vi "Generate Simulated Data v2.0.vi"(6 "Frequency":dbl, 7 "Amplitude":dbl, 8 "error in (no error)":errorcluster, 9 "Samples":i32, 10 "Total_Samples in":i64, 11 "Sample_Rate":dbl) -> (0 "error out":errorcluster, 2 "total_samples out":i64, 3 "Y":dbl[](array[numeric]))   [LabVIEW 2026, in "Acquisition.lvlib"]
uses:
  Acquisition.lvlib
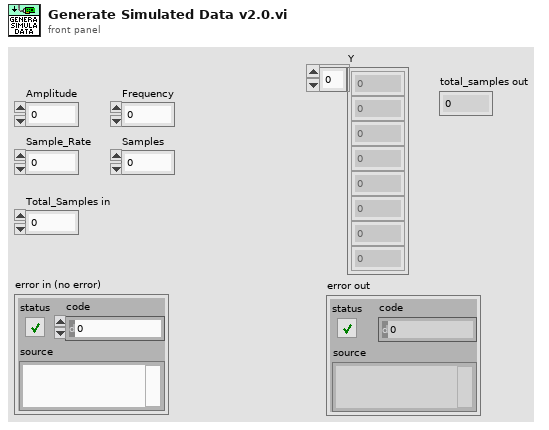
[diagram p1: front panel]
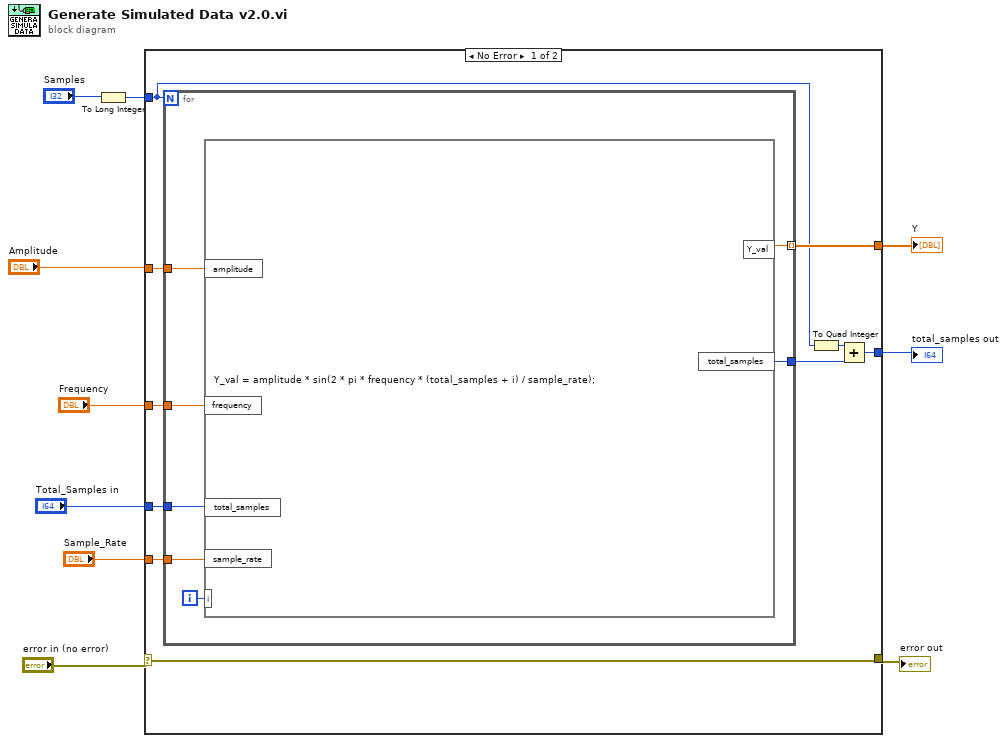
[diagram p0: block diagram]
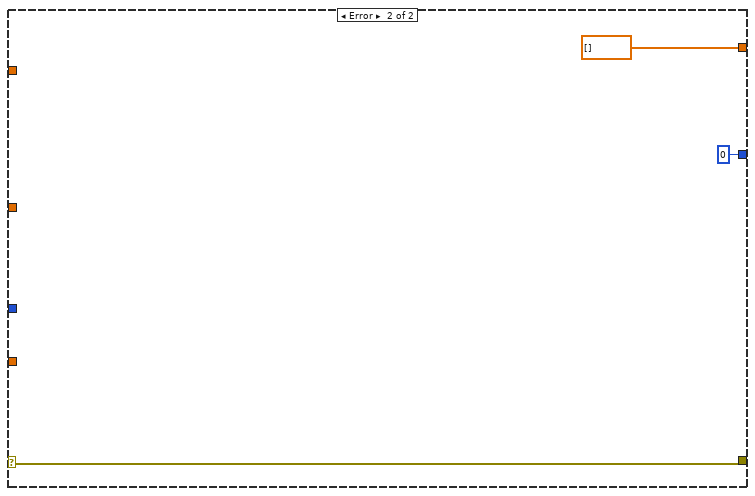
[diagram p2: hidden frame]
diagram:
  n1 = To Long Integer(number="Samples") -> (32bit integer=w2:i32)
  n2 = case shown="No Error" "error in (no error)" {
    selector: "error in (no error)" -> [w16 w30]
    tunnel: "Sample_Rate" -> [w20 _]
    tunnel: "Total_Samples in" -> [w19 _]
    tunnel: "Amplitude" -> [w18 _]
    tunnel: "Frequency" -> [w17 _]
    tunnel: [w16 w30] -> w5
    tunnel: [w15 dbl[] []] -> w4
    tunnel: w2 -> [w12 _]
    tunnel: [w11 i64 0] -> w1
    frame No Error {
      n3 = for {
        N: w12 -> [_]
        tunnel: w20 -> [w27]
        tunnel: w19 -> [w26]
        tunnel: w18 -> [w25]
        tunnel: w17 -> [w24]
        tunnel: [w23] -> w15 mode=indexing
        tunnel: [w21] -> w14
        i -> [w22]
        n4 = formula code="Y_val = amplitude * sin(2 * pi * frequency * (total_samples + i) / sample_rate);"("frequency"=w24, "amplitude"=w25, "sample_rate"=w27, "total_samples"=w26, "i"=w22) -> ("Y_val"=w23:dbl, "total_samples"=w21:i64)
      }
      n5 = To Quad Integer(1:w12) -> (0:w13:i64)
      n6 = Add(x=w13, y=w14) -> (x+y=w11:i64)
    }
    frame Error {
    }
  }
  "error out" <- w5
  "Y" <- w4
  "total_samples out" <- w1
